vi "Set Osc Channel Range.vi"(8 "error in (no error)":errorcluster, 9 "maxmv":i32, 10 "minmv":i32, 11 "channel":i32) -> (0 "error out":errorcluster, 3 "function return":i32)   [LabVIEW 2023, in "vmmsolib.lvlib"]
doc: "DLL_API int WINAPI SetOscChannelRange(int channel, int minmv, int maxmv);"
uses:
  vmmsolib.lvlib
  vmmso.dll
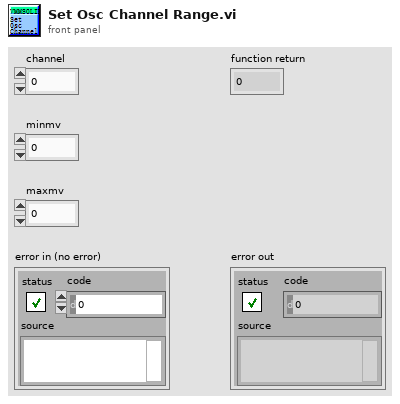
[diagram p1: front panel]
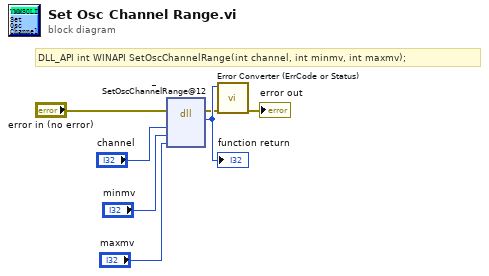
[diagram p0: block diagram]
diagram:
  # "DLL_API int WINAPI SetOscChannelRange(int channel, int minmv, int maxmv);"
  n1 = dll-call lib="D:/VmMsoSDK/demo-Labview/2023/vmmsolib/vmmso.*" fn="_SetOscChannelRange@12"(error in="error in (no error)", "channel"="channel", "minmv"="minmv", "maxmv"="maxmv") -> (error out=w2:errorcluster, w7:i32)  [unwired: 5 in, 1 out]
  "function return" <- w7
  n2 = call "Error Converter (ErrCode or Status).vi"("error in (no error)"=w2, "error code"=w7) -> ("error out"=→"error out":errorcluster)  [unwired: 9 in]
